vi "Convert to JSON.vi"(8 "error in (no error)":errorcluster, 9 "# of Objects (-1 : All)":i32=255, 10 "JSON Object (empty)":string, 11 "CBOR Hex":string) -> (0 "error out":errorcluster, 2 "CBOR Hex Out":string, 3 "<JSON Object>":string)   [LabVIEW 2020, in "CBOR.lvlib"]
uses:
  CBOR.lvlib
  <vilib>/JDP Science/JSONtext/Get all Object Items.vi
  <vilib>/JDP Science/JSONtext/JSONtext.lvlib
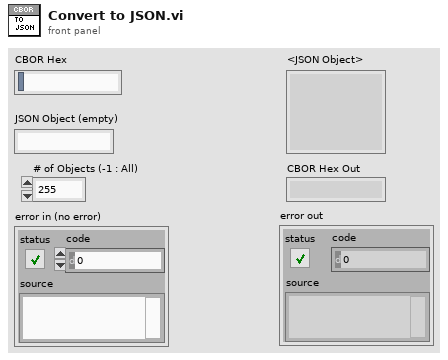
[diagram p1: front panel]
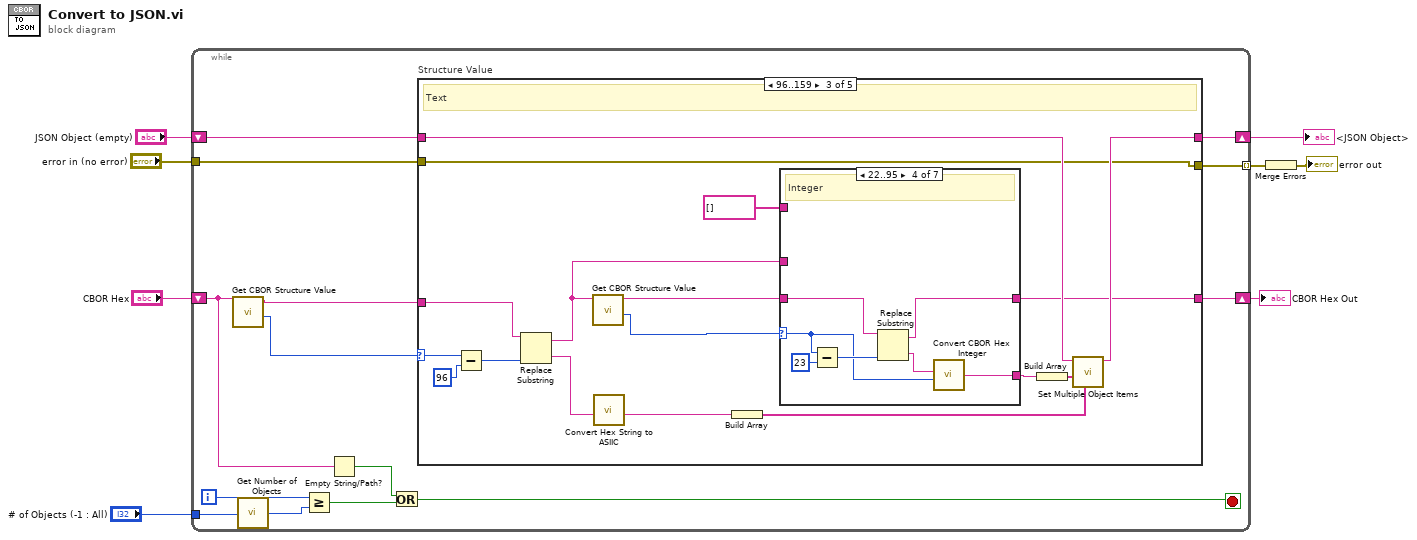
[diagram p0: block diagram]
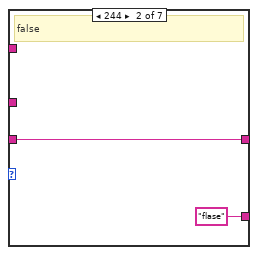
[diagram p5: hidden frame]
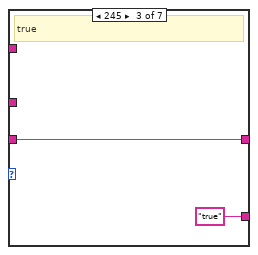
[diagram p6: hidden frame]
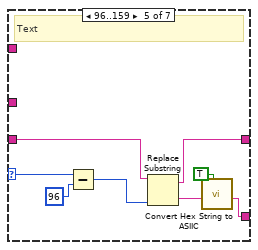
[diagram p7: hidden frame]
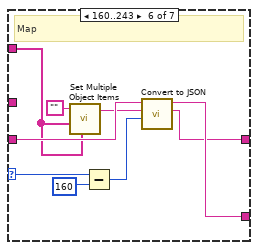
[diagram p8: hidden frame]
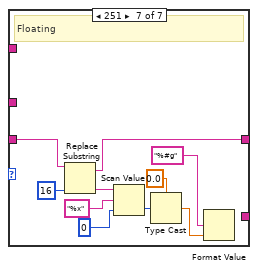
[diagram p9: hidden frame]
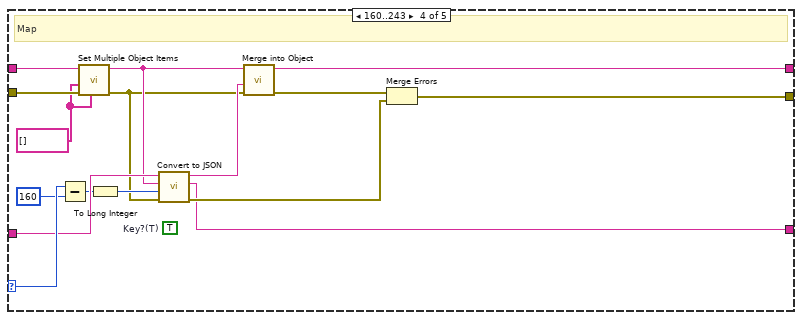
[diagram p10: hidden frame]
diagram:
  n1 = while {
    tunnel: "error in (no error)" -> [w21]
    shift-right: [w20] -> w5
    shift-left: "JSON Object (empty)" -> [w22]
    shift-right: [w19] -> w2
    shift-left: "CBOR Hex" -> [w11]
    tunnel: [w18] -> w4 mode=indexing
    tunnel: "# of Objects (-1 : All)" -> [w13]
    i -> [w14]
    stop <- w15 stop-if-true
    n2 = call "Get CBOR Structure Value.vi"("CBOR Hex"=w11) -> ("Structure Value"=w9:u8, "Remaining Data"=w10:string)  [unwired: 8 in, 1 out]
    n3 = call "Get Number of Objects.vi"("# Objects"=w13) -> ("# Objects"=w12:i32)  [unwired: 4 in]
    n4 = Greater Or Equal?(x=w14, y=w12) -> (x >= y?=w17:bool)
    n5 = Empty String/Path?(string/path=w11) -> (empty?=w16:bool)
    n6 = Or(x=w16, y=w17) -> (x .or. y?=w15:bool)
    n7 = case "Structure Value" shown="96..159" w9 {
      selector: w9 -> [_ _ w43 w99 _]
      tunnel: w10 -> [w24 _ w42 w97 _]
      tunnel: w22 -> [w25 w27 w40 w91 w101]
      tunnel: w21 -> [w23 w26 w32 w92 w100]
      tunnel: [w25 w27 w39 w94 w101] -> w20
      tunnel: [w24 _ w34 w84 _] -> w19
      tunnel: [w23 w26 w32 w85 w100] -> w18
      frame 0, Default {
      }
      frame 22..95 {
        # "Integer"
      }
      frame 96..159 {
        # "Text"
        n8 = Subtract(x=w43, y=u8 96 ("x")) -> (x-y=w28:u8)
        n9 = Replace Substring(2:w28, 5:w42) -> (0:w41:string, 1:w31:string)  [unwired: 2 in]
        n10 = call "Get CBOR Structure Value.vi"("CBOR Hex"=w31) -> ("Structure Value"=w29:u8, "Remaining Data"=w30:string)  [unwired: 8 in, 1 out]
        n11 = call "Convert Hex String to ASIIC.vi"("Hex"=w41) -> ("ASIIC"=w38:string)  [unwired: 10 in]
        n12 = Build Array(w38) -> (w37:string[])
        n13 = case shown="22..95" w29 {
          selector: w29 -> [_ _ _ w51 w63 w72 _]
          tunnel: w31 -> [_ _ _ _ _ _ _]
          tunnel: w30 -> [w45 w47 w49 w55 w62 w69 w83]
          tunnel: [_ "flase" "true" w50 w59 w70 _] -> w36
          tunnel: [w45 w47 w49 w56 w58 w65 w82] -> w34
          tunnel: string[] [] ("JSON Items") -> [_ _ _ _ _ w67 _]
          frame Default {
          }
          frame 244 {
            # "false"
          }
          frame 245 {
            # "true"
          }
          frame 22..95 {
            # "Integer"
            n14 = Subtract(x=w51, y=u8 23) -> (x-y=w53:u8)
            n15 = Replace Substring(2:w53, 5:w55) -> (0:w52:string, 1:w56:string)  [unwired: 2 in]
            n16 = call "Convert CBOR Hex Integer.vi"("Structure"=w51, "CBOR Hex"=w52) -> ("{Integer}"=w50:string)  [unwired: 2 in]
          }
          frame 96..159 {
            # "Text"
            n17 = Subtract(x=w63, y=u8 96 ("x")) -> (x-y=w57:u8)
            n18 = Replace Substring(2:w57, 5:w62) -> (0:w61:string, 1:w58:string)  [unwired: 2 in]
            n19 = call "Convert Hex String to ASIIC.vi"("Key? (T)"=TRUE, "Hex"=w61) -> ("ASIIC"=w59:string)  [unwired: 9 in]
          }
          frame 160..243 {
            # "Map"
            n20 = call <vilib>:"Set Multiple Object Items.vi"("Item Names"=w67, "JSON Items"=w67, "JSON"="") -> ("<JSON>"=w68:string)  [unwired: 6 in, 1 out]
            n21 = Subtract(x=w72, y=u8 160) -> (x-y=w73:u8)
            n22 = call "Convert to JSON.vi"("# of Objects (-1 : All)"=w73, "JSON Object (empty)"=w68, "CBOR Hex"=w69) -> ("CBOR Hex Out"=w65:string, "<JSON Object>"=w70:string)  [unwired: 6 in, 1 out]
          }
          frame 251 {
            # "Floating"
            n23 = Replace Substring(2:16 ("length (len. of substring)"), 5:w83) -> (0:w78:string, 1:w82:string)  [unwired: 2 in]
            n24 = Scan Value(string=w78, format string="%x", default (0 dbl)=u64 0) -> (value=w76:u64)  [unwired: 1 out]
            n25 = Type Cast(type=0.0, x=w76) -> (*(type *) &x=w75:dbl)
            n26 = Format Value(format string="%#g", value (0)=w75) -> ()  [unwired: 1 in, 1 out]
          }
        }
        n27 = Build Array(w36) -> (w35:string[])
        n28 = call <vilib>:"Set Multiple Object Items.vi"("Item Names"=w37, "JSON Items"=w35, "JSON"=w40) -> ("<JSON>"=w39:string)  [unwired: 6 in, 1 out]
      }
      frame 160..243 {
        w86 = string[] [] ("JSON Items")
        (unwired) TRUE  # Key?(T)
        # "Map"
        n29 = Subtract(x=w99, y=u32 160) -> (x-y=w96:u32)
        n30 = call <vilib>:"Set Multiple Object Items.vi"("Item Names"=w86, "error in (no error)"=w92, "JSON Items"=w86, "JSON"=w91) -> ("error out"=w89:errorcluster, "<JSON>"=w90:string)  [unwired: 5 in]
        n31 = To Long Integer(number=w96) -> (32bit integer=w95:i32)
        n32 = call "Convert to JSON.vi"("error in (no error)"=w89, "# of Objects (-1 : All)"=w95, "JSON Object (empty)"=w90, "CBOR Hex"=w97) -> ("error out"=w87:errorcluster, "CBOR Hex Out"=w84:string, "<JSON Object>"=w93:string)  [unwired: 5 in]
        n33 = call <vilib>:"Merge into Object.vi"("error in (no error)"=w89, "JSON Object to Merge"=w93, "JSON"=w90) -> ("error out"=w88:errorcluster, "<JSON>"=w94:string)  [unwired: 6 in]
        n34 = Merge Errors(w88, w87) -> (w85:errorcluster)
      }
      frame 251 {
        # "Floating"
      }
    }
  }
  "<JSON Object>" <- w5
  "CBOR Hex Out" <- w2
  n35 = Merge Errors(w4) -> (→"error out":errorcluster)
